vi "MW100 General Start.vi"(8 "error in (no error)":errorcluster, 11 "MW100 Input":refnum<visa-resource-name>) -> (0 "error out":errorcluster, 3 "MW100 Output":refnum<visa-resource-name>="MW100")   [LabVIEW 2023]
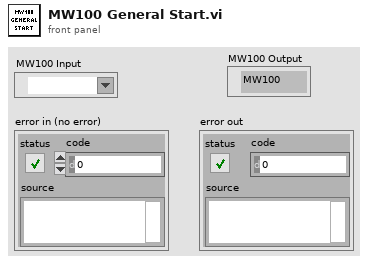
[diagram p1: front panel]
types:
  T1 = enum16{"Computation Start", "Computation stop", "Reset Computation", "Clear Computation"}
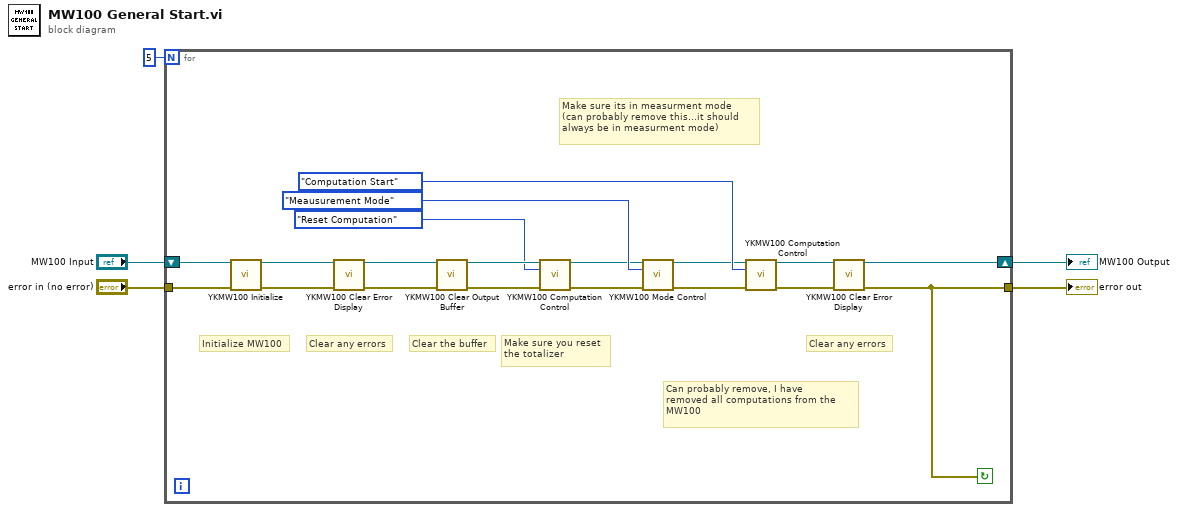
[diagram p0: block diagram]
diagram:
  n1 = for {
    N: 5 -> [_]
    shift-right: [w8] -> w3
    shift-left: "MW100 Input" -> [w23]
    tunnel: "error in (no error)" -> [w24]
    tunnel: [w6] -> w2
    stop <- w6 continue-if-true
    # "Clear any errors"
    # "Make sure you reset\nthe totalizer"
    # "Can probably remove, I have \nremoved all computations from the \nMW100"
    # "Make sure its in measurment mode\n(can probably remove this...it should \nalways be in measurment mode)"
    # "Clear the buffer"
    # "Clear any errors"
    # "Initialize MW100"
    n2 = call "YKMW100 Initialize.vi"("VISA session (TCPIP::)"=w23, "error in (no error)"=w24) -> ("dup VISA session"=w22:refnum<visa-resource-name>, "error out"=w19:errorcluster)  [unwired: 12 in]
    n3 = call "YKMW100 Clear Error Display.vi"("VISA session"=w22, "error in (no error)"=w19) -> ("dup VISA session"=w21:refnum<visa-resource-name>, "error out"=w20:errorcluster)  [unwired: 10 in, 2 out]
    n4 = call "YKMW100 Clear Output Buffer.vi"("VISA session"=w21, "error in (no error)"=w20) -> ("dup VISA session"=w12:refnum<visa-resource-name>, "error out"=w14:errorcluster)  [unwired: 12 in]
    n5 = call "YKMW100 Computation Control.vi"("VISA session"=w12, "Mode"=T1."Reset Computation", "error in (no error)"=w14) -> ("dup VISA session"=w11:refnum<visa-resource-name>, "error out"=w13:errorcluster)  [unwired: 11 in]
    n6 = call "YKMW100 Mode Control.vi"("VISA session"=w11, "Model"=enum16{"Meausurement Mode", "Setting Mode"}."Meausurement Mode", "error in (no error)"=w13) -> ("dup VISA session"=w15:refnum<visa-resource-name>, "error out"=w16:errorcluster)  [unwired: 11 in]
    n7 = call "YKMW100 Computation Control.vi"("VISA session"=w15, "Mode"=T1."Computation Start", "error in (no error)"=w16) -> ("dup VISA session"=w9:refnum<visa-resource-name>, "error out"=w7:errorcluster)  [unwired: 11 in]
    n8 = call "YKMW100 Clear Error Display.vi"("VISA session"=w9, "error in (no error)"=w7) -> ("dup VISA session"=w8:refnum<visa-resource-name>, "error out"=w6:errorcluster)  [unwired: 10 in, 2 out]
  }
  "error out" <- w2
  "MW100 Output" <- w3
